vi "Convert RPC Error to LabVIEW Error.vi"(9 "JSON Value in":refnum<class "JSON Value.lvclass">, 11 "RPC Error Code":i32) -> (2 "error out":errorcluster)   [LabVIEW 2016, in "JSONRPC Client.lvclass"]
uses:
  JSONRPC Client.lvclass
  <vilib>/NI/JSON Support for LabVIEW/JSON Value/JSON Value.lvclass
  <vilib>/NI/JSON Support for LabVIEW/JSON Value/Object/Get Value/Get Value (Numeric).vi
  <vilib>/NI/JSON Support for LabVIEW/JSON Value/Object/Get Value/Get Value (String).vi
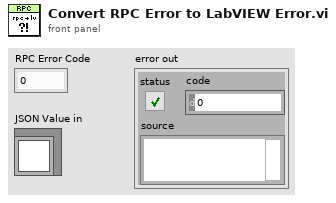
[diagram p1: front panel]
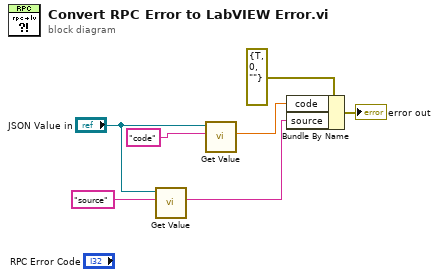
[diagram p0: block diagram]
diagram:
  n1 = call-poly <vilib>:"Get Value.vi"("key"="source", "JSON Value in"="JSON Value in") -> ("value"=w1:string)  [unwired: 8 in, 1 out]
  n2 = call-poly <vilib>:"Get Value.vi"("key"="code" ("Parameter Name"), "JSON Value in"="JSON Value in") -> ("value"=w2:dbl)  [unwired: 8 in, 1 out]
  n3 = Bundle By Name(cluster=errorcluster {"status"=TRUE, "code"=0, "source"=""} ("error constant"), "code"=w2, "source"=w1) -> (→"error out":errorcluster)
